vi "Control - Throttle Mass Flow Calc.vi"(11 "Inputs":T1={"Valve Inlet Pressure [kPa]"=0.0, "Valve Outlet Pressure [kPa]"=0.0, "Valve Inlet Temp [C]"=0.0, "Valve Position [%Open]"=0.0, "Valve Diameter [m]"=0.0, "R - Gas constant [J/kg-K]"=289.0, "k - Ratio of specific heats"=1.4, "Valve Cd"=0.0}) -> (3 "Throttle Mass Flow [kg/hr]":sgl)   [LabVIEW 2015, in "ECS-RT.lvlib"]
uses:
  ECS-RT.lvlib
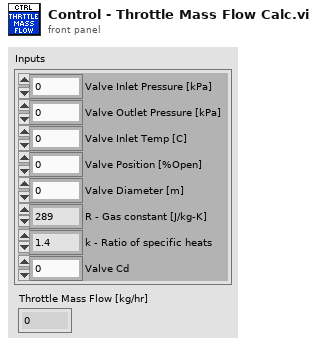
[diagram p1: front panel]
types:
  T1 = cluster{"Valve Inlet Pressure [kPa]":sgl, "Valve Outlet Pressure [kPa]":sgl, "Valve Inlet Temp [C]":sgl, "Valve Position [%Open]":sgl, "Valve Diameter [m]":sgl, "R - Gas constant [J/kg-K]":sgl, "k - Ratio of specific heats":sgl, "Valve Cd":sgl}
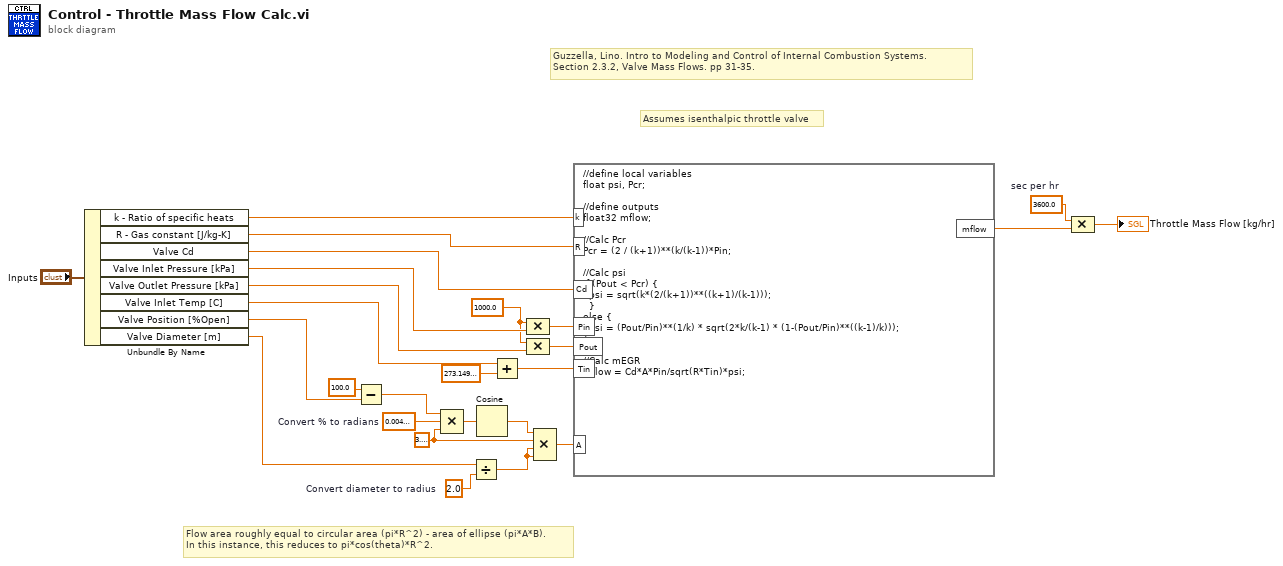
[diagram p0: block diagram]
diagram:
  w3 = sgl 1000.0 ("y")
  w15 = sgl 3600.0  # sec per hr
  w22 = 3.141592653589793
  w25 = sgl 2.0  # Convert diameter to radius
  w26 = sgl 0.005  # Convert % to radians
  # "Assumes isenthalpic throttle valve"
  # "Guzzella, Lino. Intro to Modeling and Control of Internal Combustion Systems.  \nSection 2.3.2, Valve Mass Flows. pp 31-35."
  # "Flow area roughly equal to circular area (pi*R^2) - area of ellipse (pi*A*B).\nIn this instance, this reduces to pi*cos(theta)*R^2."
  n1 = Unbundle By Name("Inputs") -> ("k - Ratio of specific heats"=w1:sgl, "R - Gas constant [J/kg-K]"=w2:sgl, "Valve Cd"=w13:sgl, "Valve Inlet Pressure [kPa]"=w4:sgl, "Valve Outlet Pressure [kPa]"=w5:sgl, "Valve Inlet Temp [C]"=w12:sgl, "Valve Position [%Open]"=w9:sgl, "Valve Diameter [m]"=w11:sgl)
  n2 = Subtract(x=sgl 100.0 ("y"), y=w9) -> (x-y=w8:sgl)
  n3 = Compound Arithmetic op=MULTIPLY(w8, w26, w22) -> (w24:dbl)
  n4 = Divide(x=w11, y=w25) -> (x/y=w21:sgl)
  n5 = Cosine(x=w24) -> (cos(x)=w23:dbl)
  n6 = Add(x=w12, y=sgl 273.15) -> (x+y=w19:sgl)
  n7 = Compound Arithmetic op=MULTIPLY(w3, w4) -> (w7:sgl)
  n8 = Compound Arithmetic op=MULTIPLY(w3, w5) -> (w6:sgl)
  n9 = Compound Arithmetic op=MULTIPLY(w23, w22, w21, w21) -> (w20:dbl)
  n10 = formula code="//define local variables\nfloat psi, Pcr;\n\n//define outputs\nfloat32 mflow;\n\n//Calc Pcr\nPcr = (2 / (k+1))**(k/(k-1))*Pin;\n\n//Calc psi\nif (Pout < Pcr) {\n  psi = sqrt(k*(2/(k+1))**((k+1)/(k-1)));\n  }\nelse {\n  psi = (Pout/Pin)**(1/k) * sqrt(2*k/(k-1) * (1-(Pout/Pin)**((k-1)/k)));\n}\n\n//Calc mEGR\nmflow = Cd*A*Pin/sqrt(R*Tin)*psi;"("A"=w20, "Pin"=w7, "Pout"=w6, "Cd"=w13, "R"=w2, "k"=w1, "Tin"=w19) -> ("mflow"=w17:sgl)
  n11 = Compound Arithmetic op=MULTIPLY(w15, w17) -> (→"Throttle Mass Flow [kg/hr]":sgl)
